vi "clicks.vi"(10 "planing":bool, 11 "reset":bool) -> (3 "function return":i32)   [LabVIEW 2017, in "HapticSTM.lvlib"]
doc: "extern \"C\" __declspec(dllexport) int clicks(bool reset);\nextern \"C\" __declspec(dllexport) int clicks(bool reset, bool planing);"
uses:
  HapticSTM.lvlib
  <userlib>/HapticSTM/HapticSTM.dll
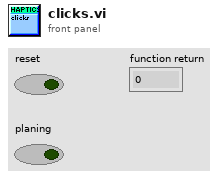
[diagram p1: front panel]
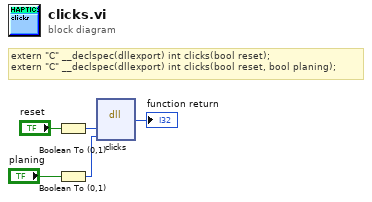
[diagram p0: block diagram]
diagram:
  # "extern \"C\" __declspec(dllexport) int clicks(bool reset);\nextern \"C\" __declspec(dllexport) int clicks(bool reset, bool planing);"
  n1 = Boolean To (0,1)(Boolean="reset") -> (0, 1=w3:i16)
  n2 = Boolean To (0,1)(Boolean="planing") -> (0, 1=w1:i16)
  n3 = dll-call lib="C:/Program Files/National Instruments/LabVIEW 2017/user.lib/HapticSTM/HapticSTM.*" fn="clicks"("reset"=w3, "planing"=w1) -> (→"function return":i32)  [unwired: 5 in, 2 out]
